vi "test_clusterWithEnums.vi"() -> ()   [LabVIEW 2020]
uses:
  _built_ppls/OpenDescriptor.lvlibp
  _built_ppls/OpenVariant.lvlibp
panel:
  out "unsigned byte array":u8[](array[numeric]) format="%.0x"
  out "type descriptor":i16[](array[numeric]) format="%04x"
  out "Value 2":variant
  out "Type":u8 format="%.0x"
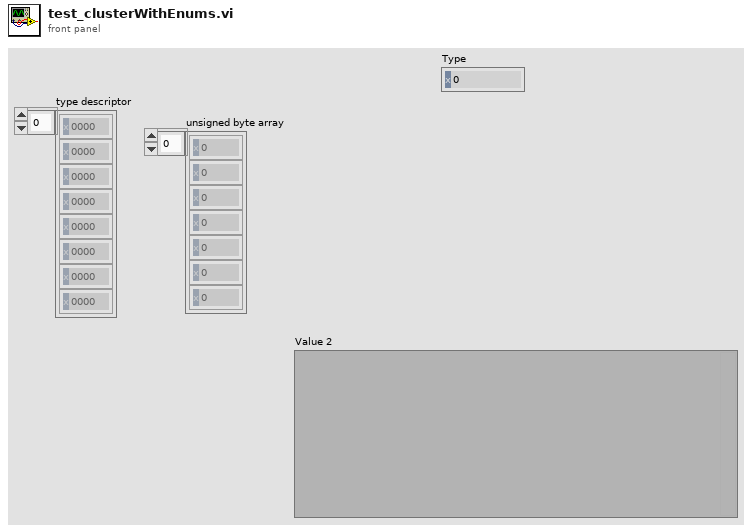
[diagram p1: front panel]
types:
  T1 = cluster{"Numeric":i8, "enum":enum8{"Item1", "Item2", "Item3"}}
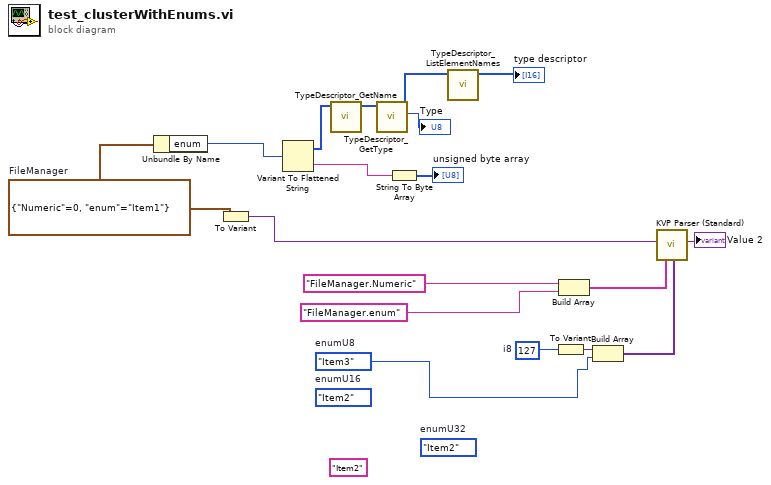
[diagram p0: block diagram]
diagram:
  (unwired) "Item2"
  (unwired) enum32{"Item1", "Item2", "Item3"}."Item2"  # enumU32
  (unwired) enum16{"Item1", "Item2", "Item3"}."Item2"  # enumU16
  w5 = enum8{"Item1", "Item2", "Item3"}."Item3"  # enumU8
  w9 = i8 127  # i8
  w11 = T1 {"Numeric"=0, "enum"=enum."Item1"}  # FileManager
  n1 = Unbundle By Name(w11) -> ("enum"=w10:enum8{"Item1", "Item2", "Item3"})
  n2 = To Variant(anything=w11) -> (Variant=w4:variant)
  n3 = Variant To Flattened String(Variant=w10) -> (data string=w13:string, 1:w18:i16[])
  n4 = call "TypeDescriptor_GetName.vi"("type descriptor"=w18) -> ("type descriptor dup"=w17:i16[])  [unwired: 8 in, 2 out]
  n5 = call "TypeDescriptor_GetType.vi"("type descriptor"=w17) -> ("Type"=→"Type":u8, "type descriptor dup"=w15:i16[])  [unwired: 9 in]
  n6 = String To Byte Array(string=w13) -> (unsigned byte array=→"unsigned byte array":u8[])
  n7 = call "TypeDescriptor_ListElementNames.vi"("type descriptor"=w15) -> ("type descriptor dup"=→"type descriptor":i16[])  [unwired: 7 in, 3 out]
  n8 = To Variant(anything=w9) -> (Variant=w8:variant)
  n9 = Build Array("FileManager.Numeric", "FileManager.enum") -> (w3:string[])
  n10 = Build Array(w8, w5) -> (w2:variant[])
  n11 = call "KVP Parser (Standard).vi"("Values"=w2, "Keys"=w3, "Default Value"=w4) -> ("Value"=→"Value 2":variant)  [unwired: 5 in, 3 out]
